vi "WD_Check.vi"(8 "error in (no error)":errorcluster, 10 "barcode 資料":cluster{"barcode A":string, "barcode B":string}, 11 "DBlink":string="Driver={ODBC Driver 17 for SQL Server};Server=localhost\\SQLEXPRESS;Database=ZDX201;UID=labview;PWD=Dsa@54137926") -> (0 "error out":errorcluster)   [LabVIEW 2019]
uses:
  <vilib>/addons/database/Connection.llb/DB Tools Open Connec (String).vi
  <vilib>/addons/database/Connection.llb/Conn Execute.vi
  <vilib>/addons/database/Recordset.llb/Rec Fetch Recordset Data (R).vi
  <vilib>/addons/database/Recordset.llb/Rec Destroy - Connection.vi
  <vilib>/addons/database/_DB Variant To Data/Database Variant To Data.xnode
  <vilib>/addons/database/NI_Database_API.lvlib
panel:
  out "查詢結果":string="Update [workplace_data] \nset  \n[barcode A] = NULL       \n  ,[barcode B] = NULL\n \n  where [workplace_name_id]= -1"
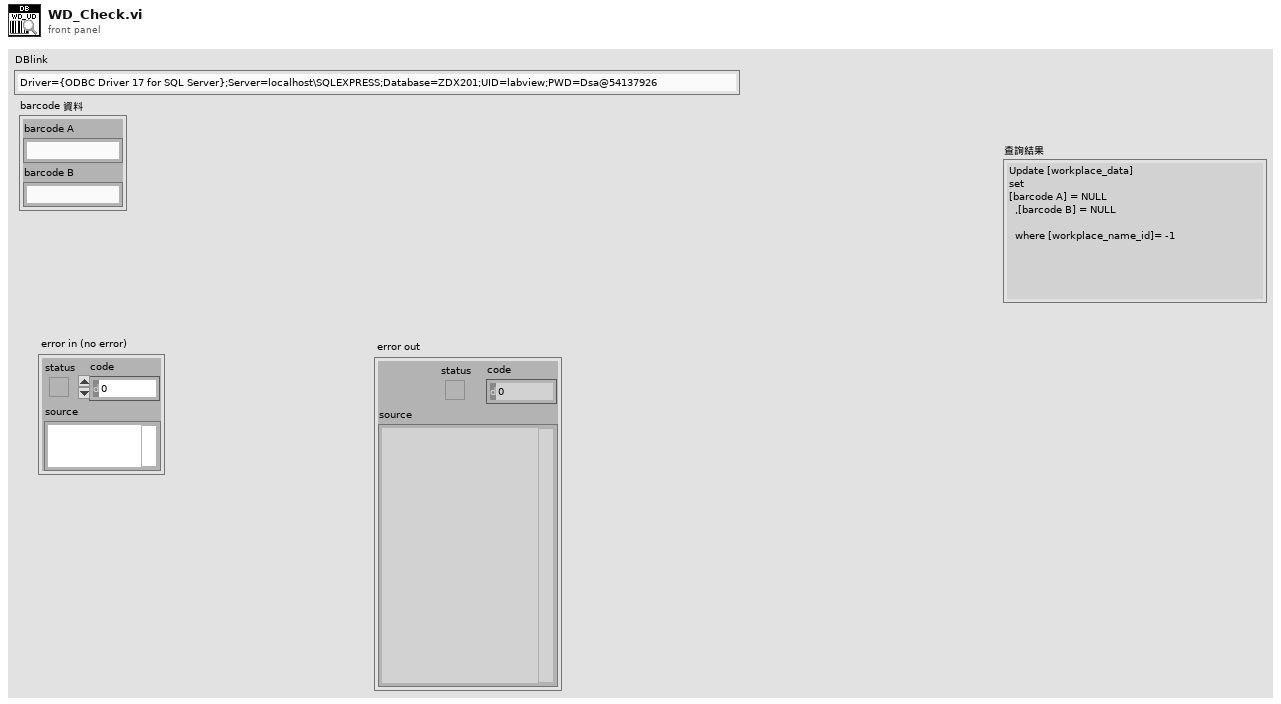
[diagram p1: front panel]
types:
  T1 = typedef "NI_Database_API.lvlib/Conn ObjectReference.ctl" = refnum<k1>
  T2 = typedef "NI_Database_API.lvlib/Rec ObjectReference.ctl" = refnum<k1>
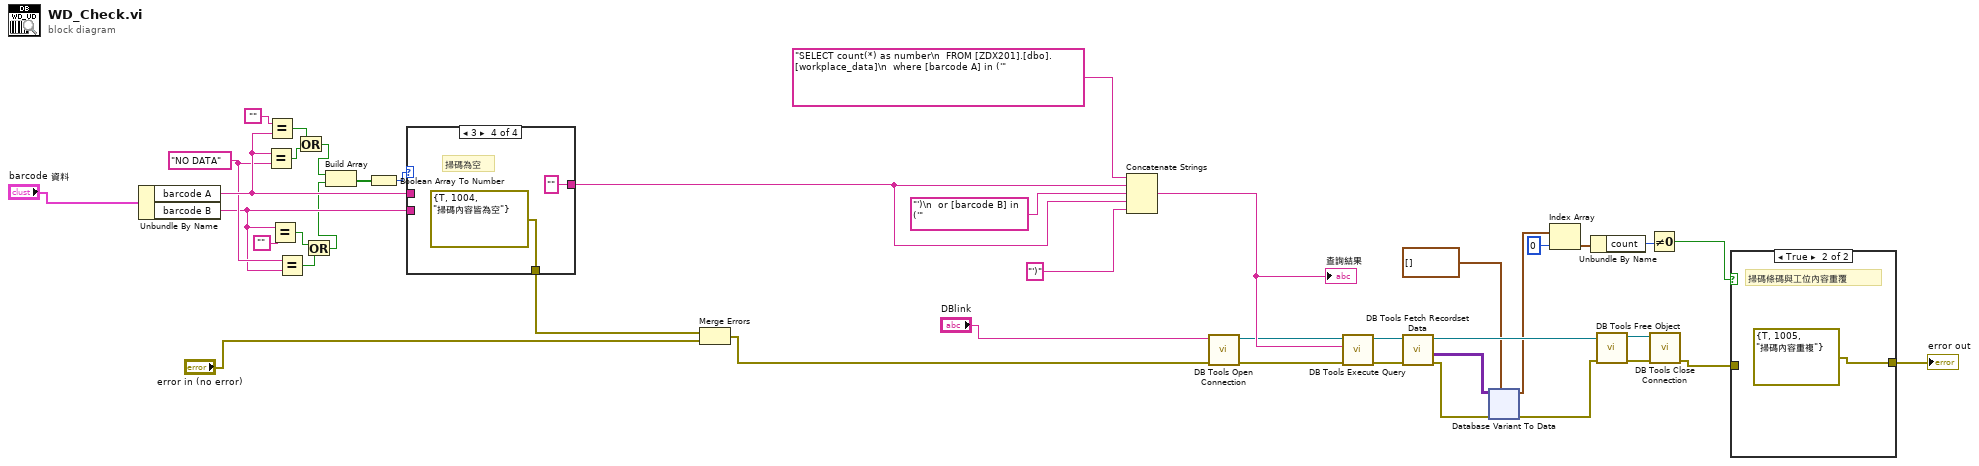
[diagram p0: block diagram]
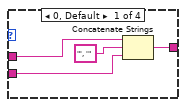
[diagram p2: hidden frame]
diagram:
  w8 = "NO DATA"
  n1 = Unbundle By Name("barcode 資料") -> ("barcode A"=w9:string, "barcode B"=w7:string)
  n2 = Equal?(x=w9, y=w8) -> (x = y?=w5:bool)
  n3 = Equal?(x="", y=w9) -> (x = y?=w6:bool)
  n4 = Equal?(x=w7, y="") -> (x = y?=w3:bool)
  n5 = Equal?(x=w8, y=w7) -> (x = y?=w2:bool)
  n6 = Or(x=w6, y=w5) -> (x .or. y?=w4:bool)
  n7 = Or(x=w3, y=w2) -> (x .or. y?=w1:bool)
  n8 = Build Array(w4, w1) -> (w14:bool[])
  n9 = Boolean Array To Number(Boolean array=w14) -> (number=w13:u32)
  n10 = case shown="3" w13 {
    tunnel: [w42 w46 w47 "" ("barcode A")] -> w26
    tunnel: w9 -> [w44 _ w47 _]
    tunnel: w7 -> [w43 w46 _ _]
    tunnel: [_ _ _ errorcluster {"status"=TRUE, "code"=1004, "source"="掃碼內容皆為空"} ("error constant")] -> w12
    frame 0, Default {
      n11 = Concatenate Strings(w44, "', '", w43) -> (w42:string)
    }
    frame 1 {
    }
    frame 2 {
    }
    frame 3 {
      # "掃碼為空"
    }
  }
  n12 = Merge Errors(w12, "error in (no error)") -> (w10:errorcluster)
  n13 = Concatenate Strings("SELECT count(*) as number\n  FROM [ZDX201].[dbo].[workplace_data]\n  where [barcode A] in ('", w26, "')\n  or [barcode B] in ('", w26, "')") -> (w41:string)
  "查詢結果" <- w41
  n14 = call-poly <vilib>:"DB Tools Open Connection.vi"("error in (no error)"=w10, "connection information"="DBlink") -> ("error out"=w32:errorcluster, "connection reference"=w33:T1)  [unwired: 6 in]
  n15 = call-poly <vilib>:"DB Tools Execute Query.vi"("error in (no error)"=w32, "SQL query"=w41, "connection reference"=w33) -> ("error out"=w35:errorcluster, "recordset reference"=w34:T2)  [unwired: 5 in]
  n16 = call-poly <vilib>:"DB Tools Fetch Recordset Data.vi"("error in (no error)"=w35, "recordset reference"=w34) -> ("error out"=w40:errorcluster, "recordset data"=w22:variant[][], "recordset reference out"=w39:T2)  [unwired: 3 in]
  n17 = xnode "Database Variant To Data"("database variant"=w22, "error in (no error)"=w40, "type"=cluster{"count":i16}[] [] ("Workplace: assemble")) -> ("data"=w24:cluster{"count":i16}[], "error out"=w38:errorcluster)
  n18 = Index Array(array=w24, index=0) -> (element=w21:cluster{"count":i16})
  n19 = Unbundle By Name(w21) -> ("count"=w20:i16)
  n20 = call-poly <vilib>:"DB Tools Free Object.vi"("error in (no error)"=w38, "recordset reference"=w39) -> ("error out"=w37:errorcluster, "connection reference"=w36:T1)  [unwired: 8 in]
  n21 = Not Equal To 0?(x=w20) -> (x != 0?=w16:bool)
  n22 = call <vilib>:"DB Tools Close Connection.vi"("error in (no error)"=w37, "connection reference"=w36) -> ("error out"=w17:errorcluster)  [unwired: 5 in]
  n23 = case shown="True" w16 {
    tunnel: w17 -> [w50 _]
    tunnel: [w50 errorcluster {"status"=TRUE, "code"=1005, "source"="掃碼內容重複"} ("error constant")] -> w15
    frame False {
    }
    frame True {
      # "掃碼條碼與工位內容重覆"
    }
  }
  "error out" <- w15
